vi "private_data.get.vi"(8 "error in (no error)":errorcluster, 11 "reqwest in":refnum<class "reqwest.lvclass">) -> (0 "error out":errorcluster, 2 "private data":T1={"Default Headers ([JSON])"=[{"header"="Content-Type", "value"="application/json"}], "Base URL"="", "Authentication"={"Username"="", "Password"=""}}, 3 "reqwest out":refnum<class "reqwest.lvclass">)   [LabVIEW 2020, in "reqwest.lvclass"]
uses:
  reqwest.lvclass
  private_data.ctl
  <vilib>/addons/_JKI.lib/REST Client/classes/REST Client/HTTP Header.ctl
  reqwest.lvclass/reqwest.ctl
  <vilib>/addons/_JKI.lib/REST Client/classes/REST Client/REST Client.lvclass
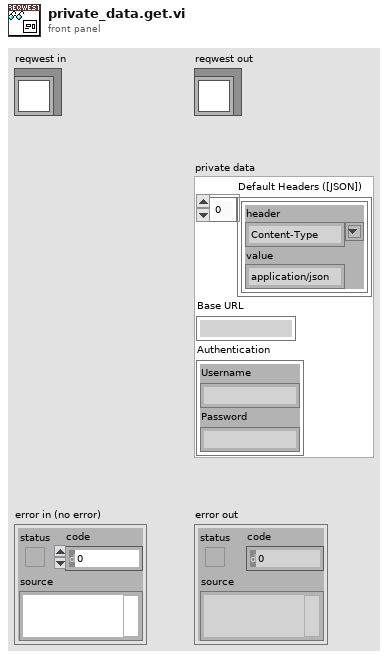
[diagram p1: front panel]
types:
  T1 = typedef "reqwest.lvclass/private_data.ctl" = cluster{"Default Headers ([JSON])":T2[], "Base URL":string, "Authentication":cluster{"Username":string, "Password":string}}
  T2 = typedef "REST Client.lvlib/REST Client.lvclass/HTTP Header.ctl" = cluster{"header":string, "value":string}
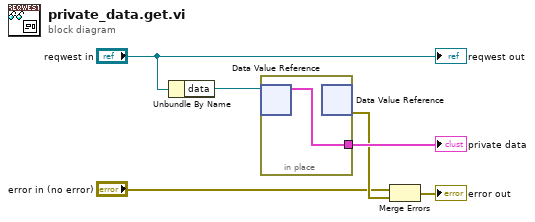
[diagram p0: block diagram]
diagram:
  n1 = Unbundle By Name("reqwest in") -> ("data"=w4:refnum<data-value>)
  n2 = in-place {
    in-place-border: [w7] -> w5
    n3 = in-place-dvr #1(w4) -> (w7:T1)  [unwired: 1 out]
    n4 = in-place-dvr #1() -> (w3:errorcluster)  [unwired: 1 in, 1 out]
  }
  "private data" <- w5
  n5 = Merge Errors("error in (no error)", w3) -> (→"error out":errorcluster)
  "reqwest out" <- "reqwest in"
